vi "svfa_Check Data Valid [Zoom] (N Ch).vi"(0 "scaled signals [EU]":waveform(dbl)[](array[waveform]), 1 "restart averaging (F)":bool, 9 "averaging parameters":T2={"averaging mode"=enum."No averaging", "weighting mode"=enum."Linear", "number of averages"=10, "linear mode"=enum."Auto restart"}, 11 "error in (no error)":errorcluster, 12 "zoom settings":T3={"frequency range"={"start frequency"=1000.0, "stop frequency"=2000.0}, "window"=1, "number of lines"=400, "% overlap"=0.0} {"% overlap" min=0.0 format="%.2f"; "number of lines" min=2; "window" items=["None ", "Hanning", "Hamming", "Blackman-Harris", "Exact Blackman", "Blackman", "Flat Top", "4 Term B-Harris ", "7 Term B-Harris", "Low Sidelobe"]; "frequency range"."stop frequency" min=0.0 format="%.2f"; "frequency range"."start frequency" min=0.0 format="%.2f"}) -> (2 "reset processing":bool, 3 "restart averaging":bool, 4 "dup scaled signals":waveform(dbl)[](array[waveform]), 6 "iterations":i32, 8 "maximum block size":i32, 10 "dup averaging parameters":T2={"averaging mode"=enum."No averaging", "weighting mode"=enum."Linear", "number of averages"=10, "linear mode"=enum."Auto restart"}, 14 "zoom FFT settings":T1={"zoom settings"={"center frequency"=-inf, "zoom"=1, "trim"=1.0}, "FFT settings"={"window"=enum."Hanning", "window size"=-1, "FFT size"=1024, "%overlap"=0.0}} {"FFT settings"."%overlap" min=0.0 max=100.0 format="%.2f"; "zoom settings"."trim" min=1.0 format="%.2f"; "zoom settings"."center frequency" format="%.2f"; "zoom settings"."zoom" min=1}, 15 "error out":errorcluster)   [LabVIEW 2017]
uses:
  <vilib>/addons/_NISVFA/_Shared subVIs/Common/svc_Check for Waveform Parameter Continuity (no state).vi
  <vilib>/addons/_NISVFA/_Shared subVIs/Common/svc_Get SV Channel Info.vi
  <vilib>/addons/_NISVFA/_Shared subVIs/Common/svc_Engineering Units to Unit Label.vi
  <vilib>/addons/_NISVFA/_Shared subVIs/Common/svc_Unit Label to Engineering Units.vi
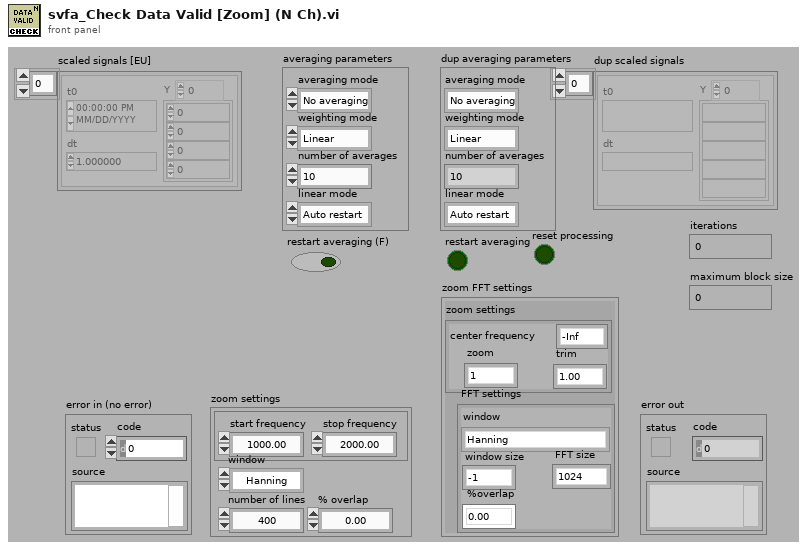
[diagram p1: front panel]
types:
  T1 = cluster{"zoom settings":cluster{"center frequency":dbl, "zoom":i32, "trim":dbl}, "FFT settings":cluster{"window":enum16{"None ", "Hanning", "Hamming", "Blackman-Harris", "Exact Blackman", "Blackman", "Flat Top", "4 Term B-Harris ", "7 Term B-Harris", "Low Sidelobe"}, "window size":i32, "FFT size":i32, "%overlap":dbl}}
  T2 = cluster{"averaging mode":enum16{"No averaging", "Vector averaging", "RMS averaging", "Peak hold"}, "weighting mode":enum16{"Linear", "Exponential"}, "number of averages":u32, "linear mode":enum16{"One shot", "Auto restart"}}
  T3 = cluster{"frequency range":cluster{"start frequency":dbl, "stop frequency":dbl}, "window":u16, "number of lines":i32, "% overlap":dbl}
  T4 = cluster{"dt equal":bool, "array length equal":bool, "number channels change":bool}
  T5 = cluster{"dt":bool, "t0 continuity":bool, "array length":bool, "channel info":bool, "name":bool}
  T6 = typedef "NI_AALPro.lvlib/windowTd.ctl" = u32
  T7 = enum16{"No averaging", "Vector averaging", "RMS averaging", "Peak hold"}
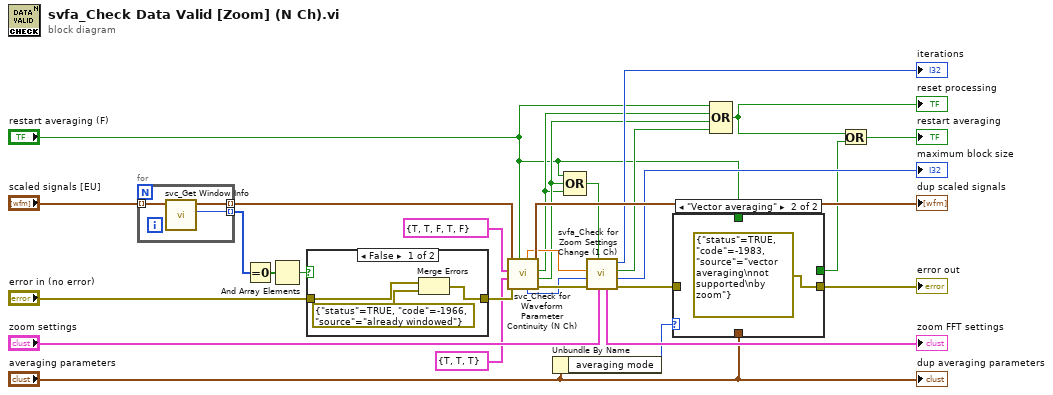
[diagram p0: block diagram]
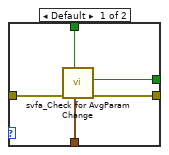
[diagram p2: hidden frame]
diagram:
  n1 = for {
    tunnel: "scaled signals [EU]" -> [w32] mode=indexing
    tunnel: [w31] -> w15 mode=indexing
    tunnel: [w30] -> w13 mode=indexing
    n2 = call <vilib>:"svc_Get Window Info.vi"("scaled signal [EU]"=w32) -> ("window"=w30:T6, "dup scaled signal [EU]"=w31:waveform(dbl))  [unwired: 6 in, 3 out]
  }
  n3 = Equal To 0?(x=w13) -> (x = 0?=w14:bool[])
  n4 = And Array Elements(Boolean array=w14) -> (logical AND=w12:bool)
  n5 = case shown="False" w12 {
    tunnel: "error in (no error)" -> [w34 w36]
    tunnel: [w35 w36] -> w11
    frame False {
      n6 = Merge Errors(w34, errorcluster {"status"=TRUE, "code"=-1966, "source"="already windowed"} ("error in 2 (no error)")) -> (w35:errorcluster)
    }
    frame True {
    }
  }
  n7 = call <vilib>:"svc_Check for Waveform Parameter Continuity (N Ch).vi"("restart averaging (F)"="restart averaging (F)", "error in (no error)"=w11, "checks for multichannel parameters"=T4 {"dt equal"=TRUE, "array length equal"=TRUE, "number channels change"=TRUE}, "checks for channel parameter change"=T5 {"dt"=TRUE, "t0 continuity"=TRUE, "array length"=FALSE, "channel info"=TRUE, "name"=FALSE}, "scaled signal(s)"=w15) -> ("error out"=w20:errorcluster, "multichannel parameter changed"=w10:bool, "waveform parameter changed"=w9:bool, "dup scaled signal(s)"=→"dup scaled signals":waveform(dbl)[], "array length"=w17:i32, "dt"=w16:dbl)  [unwired: 1 out]
  n8 = Unbundle By Name("averaging parameters") -> ("averaging mode"=w3:T7)
  n9 = Compound Arithmetic op=OR("restart averaging (F)", w10, w9) -> (w8:bool)
  n10 = call <vilib>:"svfa_Check for Zoom Settings Change (1 Ch).vi"("zoom settings"="zoom settings", "restart averaging (F)"=w8, "error in (no error)"=w20, "array length"=w17, "dt"=w16) -> ("error out"=w19:errorcluster, "maximum block size"=→"maximum block size":i32, "zoom settings changed"=w18:bool, "iterations"=→"iterations":i32, "zoom FFT settings"=→"zoom FFT settings":T1)  [unwired: 2 in]
  n11 = case shown="\"Vector averaging\"" w3 {
    tunnel: "averaging parameters" -> [w41 _]
    tunnel: w19 -> [w40 _]
    tunnel: [w39 _] -> w7
    tunnel: "restart averaging (F)" -> [w38 _]
    tunnel: [w37 errorcluster {"status"=TRUE, "code"=-1983, "source"="vector averaging\nnot supported\nby zoom"} ("error IO")] -> w5
    frame Default {
      n12 = call <vilib>:"svfa_Check for AvgParam Change.vi"("averaging parameters"=w41, "restart averaging (F)"=w38, "error in (no error)"=w40) -> ("error out"=w37:errorcluster, "parameter has changed"=w39:bool)  [unwired: 7 in]
    }
    frame "Vector averaging" {
    }
  }
  "error out" <- w5
  n13 = Compound Arithmetic op=OR("restart averaging (F)", w9, w10, w18) -> (w21:bool)
  "reset processing" <- w21
  n14 = Or(x=w21, y=w7) -> (x .or. y?=→"restart averaging":bool)
  "dup averaging parameters" <- "averaging parameters"
